vi "Get StringConstant from VI.vi"(8 "error in (no error)":errorcluster, 11 "VI in":refnum<vi>) -> (0 "error out":errorcluster, 3 "StringConstant out":refnum<vi>)   [LabVIEW 2020]
uses:
  <vilib>/Utility/traverseref.llb/TRef TravTarget.ctl
  <vilib>/Utility/traverseref.llb/VI Scripting - Traverse.lvlib
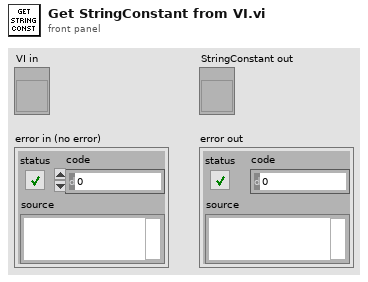
[diagram p1: front panel]
types:
  T1 = typedef "TRef TravTarget.ctl" = enum16{"FP", "BD", "Other"}
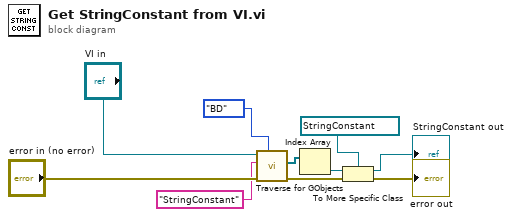
[diagram p0: block diagram]
diagram:
  n1 = call <vilib>:"Traverse for GObjects.vi"("Traverse Target"=TRef_TravTarget."BD", "error in (no error)"="error in (no error)", "Class Name"="StringConstant", "VI Refnum"="VI in") -> ("error out"=w7:errorcluster, "References"=w3:refnum<vi>[])  [unwired: 4 in, 2 out]
  n2 = Index Array(array=w3) -> (element=w5:refnum<vi>)  [unwired: 1 in]
  n3 = To More Specific Class(target class=refnum<vi> refnum ("StrCnst Refnum"), reference=w5, error in=w7) -> (specific class reference=→"StringConstant out":refnum<vi>, error out=→"error out":errorcluster)
